vi "show2.vi"() -> (2 "Picture1":picture)   [LabVIEW 2020]
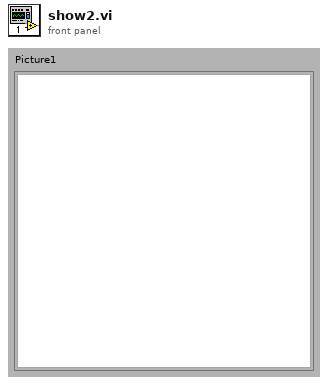
[diagram p1: front panel]
types:
  T1 = typedef "imagedata.ctl" = cluster{"image type":i32, "image depth":i32, "image":u8[], "mask":u8[], "colors":u32[], "Rectangle":cluster{"left":i16, "top":i16, "right":i16, "bottom":i16}}
  T2 = cluster{u16, u8, "image data":T1, u8[], "Array 2":u32[], cluster{i16, i16, u16, u16}}
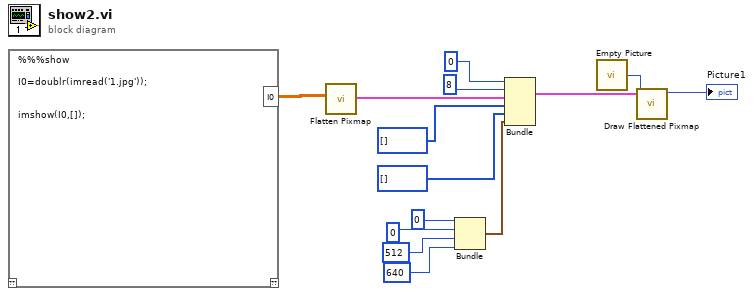
[diagram p0: block diagram]
diagram:
  n1 = script code="%%%show\n\nI0=doublr(imread('1.jpg'));\n\n\nimshow(I0,[]);"() -> ("I0"=w3:dbl[][])  [unwired: 1 in, 1 out]
  n2 = call <vilib>:"Flatten Pixmap.vi"("8-bit pixmap"=w3) -> ("image data"=w4:T1)  [unwired: 10 in]
  n3 = Bundle(i16 0, i16 0, u16 640, u16 512) -> (w11:cluster{i16, i16, u16, u16})  [unwired: 1 in]
  n4 = Bundle(u16 0, u8 8, "image data"=w4, u8[] [], "Array 2"=u32[] [], w11) -> (w2:T2)  [unwired: 1 in]
  n5 = call "Empty Picture"() -> ("empty picture"=w14:picture)
  n6 = call <vilib>:"Draw Flattened Pixmap.vi"("image data"=w2, "picture"=w14) -> ("new picture"=→"Picture1":picture)  [unwired: 7 in]
